vi "18-ReplaceRightExplode.vi"(10 "Right Explosion":u64, 11 "Right Snailfish Number in":string) -> (3 "Right Snailfish Number out":string)   [LabVIEW 2019, in "18.lvlib"]
uses:
  18.lvlib
  <vilib>/regexp/Match Regular Expression.xnode
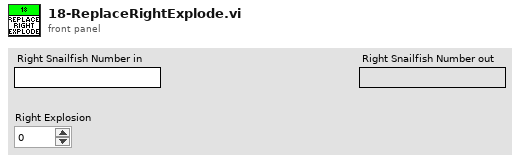
[diagram p1: front panel]
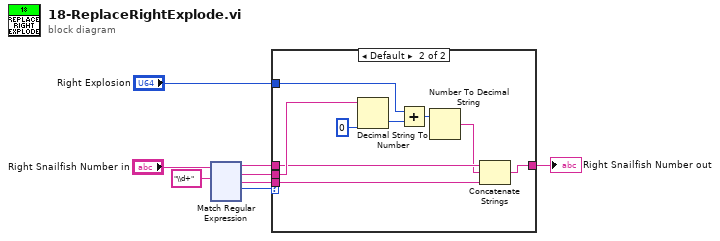
[diagram p0: block diagram]
diagram:
  n1 = xnode "Match Regular Expression"("input string"="Right Snailfish Number in", "regular expression"="\\d+") -> ("before match"=w6:string, "whole match"=w4:string, "after match"=w5:string, "offset past match"=w7:i32)  [unwired: 4 in, 1 out]
  n2 = case shown="Default" w7 {
    tunnel: "Right Explosion" -> [_ w17]
    tunnel: w6 -> [w9 w13]
    tunnel: w5 -> [_ w11]
    tunnel: w4 -> [_ w14]
    tunnel: [w9 w10] -> w1
    frame -1 {
    }
    frame Default {
      n3 = Decimal String To Number(string=w14, default (0L)=u64 0 ("default (0 I32)")) -> (number=w18:u64)  [unwired: 1 in, 1 out]
      n4 = Add(x=w17, y=w18) -> (x+y=w15:u64)
      n5 = Number To Decimal String(number=w15) -> (decimal integer string=w12:string)  [unwired: 1 in]
      n6 = Concatenate Strings(w13, w12, w11) -> (w10:string)
    }
  }
  "Right Snailfish Number out" <- w1
